vi "scale output.vi"(1 "Raw waveform":waveform(dbl)[](array[waveform]) caption="wfm", 2 "wfm info":T1(array[cluster]) {"reserved2" format="%.2f"; "reserved1" format="%.2f"; "offset" format="%^.3e"; "gain" format="%^.3e"; "xIncrement" format="%^.3e"; "relativeInitialX" format="%^.3e"; "absoluteInitialX" format="%^.3e"}) -> (0 "Scaled waveform":waveform(dbl)[](array[waveform]))   [LabVIEW 2018]
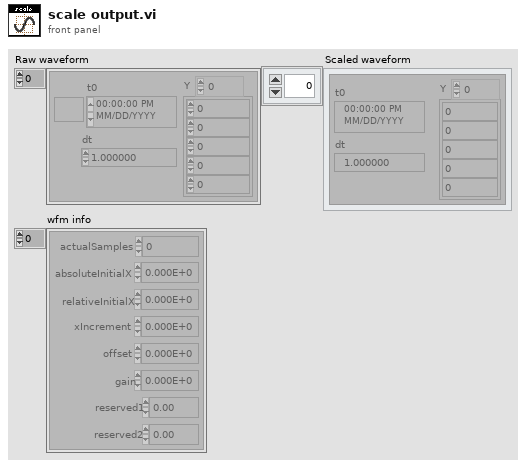
[diagram p1: front panel]
types:
  T1 = cluster{"actualSamples":i32, "absoluteInitialX":dbl, "relativeInitialX":dbl, "xIncrement":dbl, "offset":dbl, "gain":dbl, "reserved1":dbl, "reserved2":dbl}[]
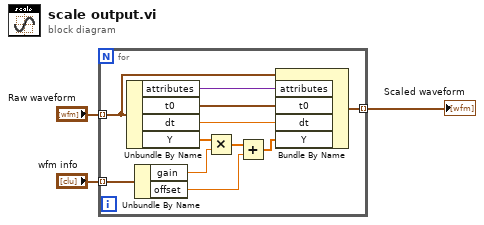
[diagram p0: block diagram]
diagram:
  n1 = for {
    tunnel: "Raw waveform" -> [w4] mode=indexing
    tunnel: "wfm info" -> [w14] mode=indexing
    tunnel: [w5] -> w1 mode=indexing
    n2 = Unbundle By Name(w4) -> ("attributes"=w9:variant, "t0"=w8:timestamp, "dt"=w7:dbl, "Y"=w10:dbl[])
    n3 = Unbundle By Name(w14) -> ("gain"=w13:dbl, "offset"=w11:dbl)
    n4 = Multiply(x=w10, y=w13) -> (x*y=w12:dbl[])
    n5 = Add(x=w12, y=w11) -> (x+y=w6:dbl[])
    n6 = Bundle By Name(cluster=w4, "attributes"=w9, "t0"=w8, "dt"=w7, "Y"=w6) -> (w5:waveform(dbl))
  }
  "Scaled waveform" <- w1
